vi "Initialization.vi"(6 "PIDAdj":refnum<vi>, 8 "error in (no error)":errorcluster, 9 "ComponentsRefs":refnum<vi>[](array[refnum]), 10 "TestType":enum16{"Normal", "Stall"}(ring), 11 "TestFixPtProc in":refnum<class "TestFixPtProc.lvclass">) -> (0 "error out":errorcluster, 3 "TestFixPtProc out":refnum<class "TestFixPtProc.lvclass">)   [LabVIEW 2024, in "TestFixPtActor.lvlib" / "TestFixPtProc.lvclass"]
uses:
  TestFixPtProc.lvclass
  TestFixPtProc.lvclass/TestFixPtProc.ctl
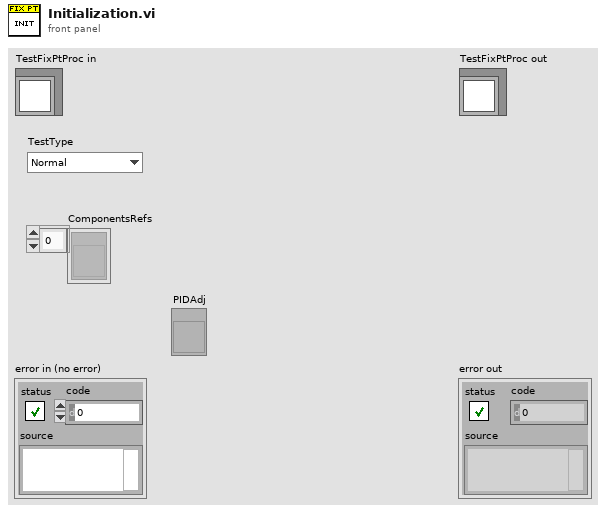
[diagram p1: front panel]
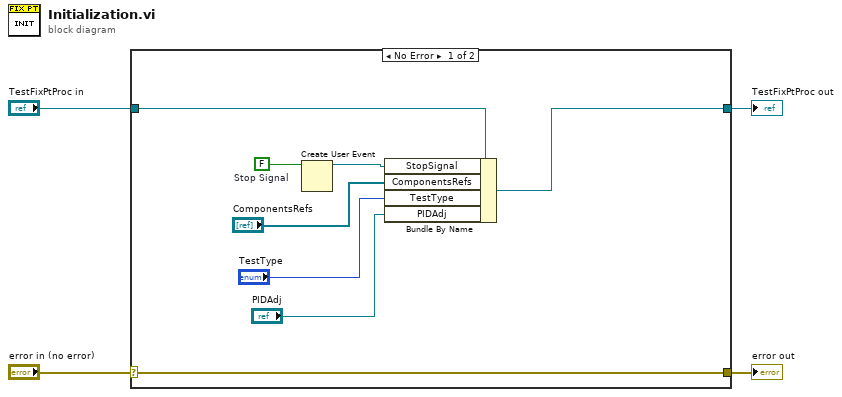
[diagram p0: block diagram]
diagram:
  n1 = case shown="No Error" "error in (no error)" {
    selector: "error in (no error)" -> [w12 w14]
    tunnel: [w12 w14] -> w3
    tunnel: [w6 w13] -> w1
    tunnel: "TestFixPtProc in" -> [w7 w13]
    frame No Error {
      w11 = FALSE  # Stop Signal
      n2 = Create User Event(user event datatype=w11) -> (user event=w10:refnum<user-event>)  [unwired: 1 in, 1 out]
      n3 = Bundle By Name(cluster=w7, "StopSignal"=w10, "ComponentsRefs"="ComponentsRefs", "TestType"="TestType", "PIDAdj"="PIDAdj") -> (w6:refnum<class "TestFixPtProc.lvclass">)
    }
    frame Error {
    }
  }
  "error out" <- w3
  "TestFixPtProc out" <- w1
